vi "Graphic Test (2D picture speed).vi"() -> ()   [LabVIEW 2024]
panel:
  out "Other computation 2 Speed (Hz)":dbl
  out "Other computation Speed (Hz)":dbl
  out "Numeric":i32
  in  "stop":bool
  out "FPS":dbl
  out "PlayingScene":picture
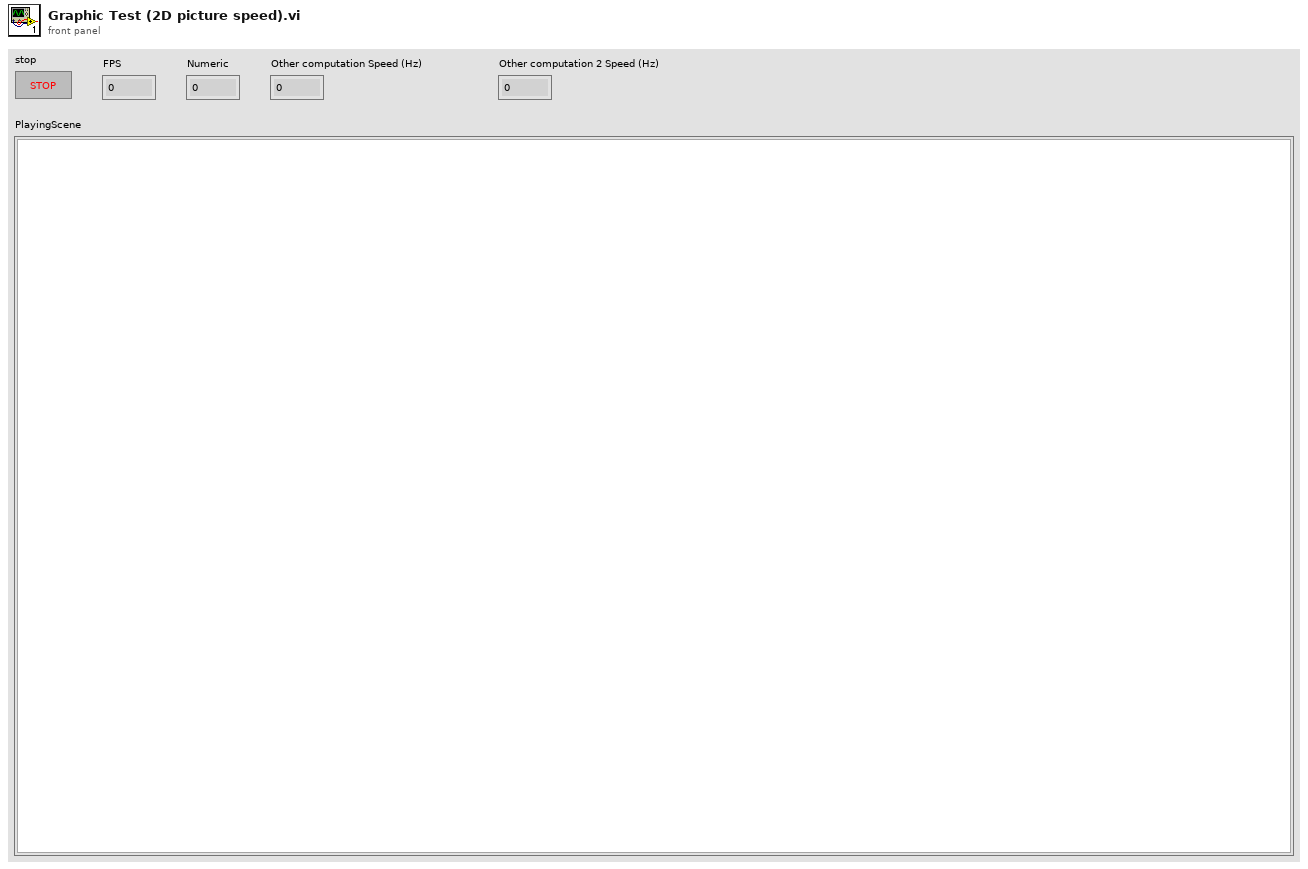
[diagram p1: front panel]
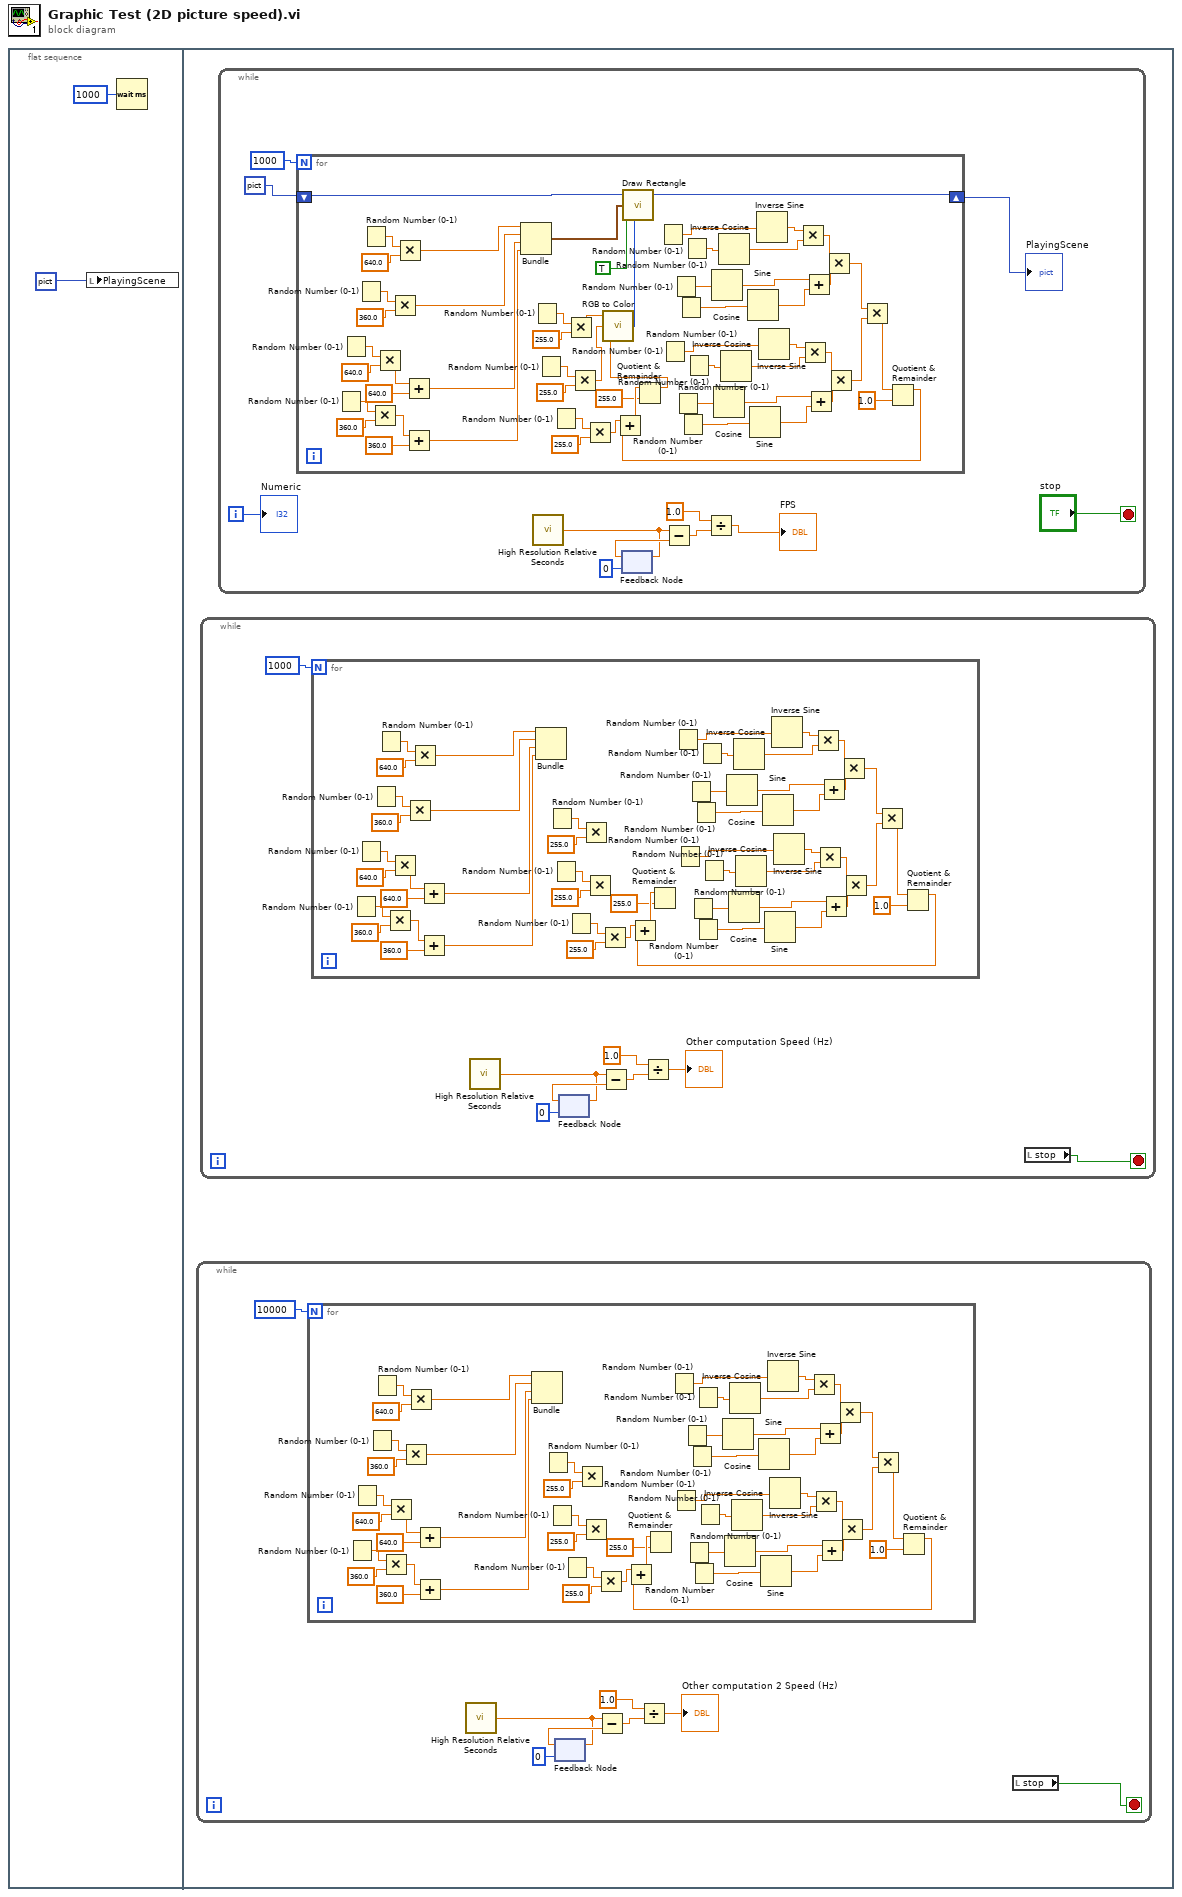
[diagram p0: block diagram]
diagram:
  n1 = flat-sequence {
    frame #0 {
      n2 = local write "PlayingScene"(picture data[5B] ("PlayingScene")) -> ()
      n3 = Wait (ms)(milliseconds to wait=u32 1000) -> ()  [unwired: 1 out]
    }
    frame #1 {
      n4 = while {
        stop <- w3 stop-if-true
        n5 = for {
          N: 10000 -> [_]
          n6 = Random Number (0-1)() -> (number: 0 to 1=w45:dbl)
          n7 = Random Number (0-1)() -> (number: 0 to 1=w47:dbl)
          n8 = Random Number (0-1)() -> (number: 0 to 1=w50:dbl)
          n9 = Random Number (0-1)() -> (number: 0 to 1=w53:dbl)
          n10 = Multiply(x=w45, y=360.0) -> (x*y=w41:dbl)
          n11 = Multiply(x=w47, y=640.0) -> (x*y=w44:dbl)
          n12 = Multiply(x=w50, y=360.0) -> (x*y=w49:dbl)
          n13 = Multiply(x=w53, y=640.0) -> (x*y=w52:dbl)
          n14 = Add(x=w44, y=640.0) -> (x+y=w43:dbl)
          n15 = Add(x=w41, y=360.0) -> (x+y=w42:dbl)
          n16 = Bundle(w52, w49, w43, w42) -> ()  [unwired: 1 in, 1 out]
          n17 = Random Number (0-1)() -> (number: 0 to 1=w59:dbl)
          n18 = Random Number (0-1)() -> (number: 0 to 1=w57:dbl)
          n19 = Random Number (0-1)() -> (number: 0 to 1=w55:dbl)
          n20 = Multiply(x=w59, y=255.0) -> ()  [unwired: 1 out]
          n21 = Multiply(x=w57, y=255.0) -> ()  [unwired: 1 out]
          n22 = Multiply(x=w55, y=255.0) -> (x*y=w26:dbl)
          n23 = Random Number (0-1)() -> (number: 0 to 1=w15:dbl)
          n24 = Random Number (0-1)() -> (number: 0 to 1=w30:dbl)
          n25 = Random Number (0-1)() -> (number: 0 to 1=w14:dbl)
          n26 = Random Number (0-1)() -> (number: 0 to 1=w29:dbl)
          n27 = Random Number (0-1)() -> (number: 0 to 1=w16:dbl)
          n28 = Random Number (0-1)() -> (number: 0 to 1=w31:dbl)
          n29 = Random Number (0-1)() -> (number: 0 to 1=w23:dbl)
          n30 = Random Number (0-1)() -> (number: 0 to 1=w38:dbl)
          n31 = Cosine(x=w14) -> (cos(x)=w20:dbl)
          n32 = Cosine(x=w29) -> (cos(x)=w35:dbl)
          n33 = Inverse Cosine(1:w23) -> (0:w21:dbl)
          n34 = Inverse Cosine(1:w38) -> (0:w36:dbl)
          n35 = Sine(x=w16) -> (sin(x)=w19:dbl)
          n36 = Sine(x=w31) -> (sin(x)=w34:dbl)
          n37 = Inverse Sine(1:w15) -> (0:w22:dbl)
          n38 = Inverse Sine(1:w30) -> (0:w37:dbl)
          n39 = Multiply(x=w22, y=w21) -> (x*y=w18:dbl)
          n40 = Multiply(x=w37, y=w36) -> (x*y=w33:dbl)
          n41 = Add(x=w20, y=w19) -> (x+y=w17:dbl)
          n42 = Add(x=w35, y=w34) -> (x+y=w32:dbl)
          n43 = Multiply(x=w18, y=w17) -> (x*y=w13:dbl)
          n44 = Multiply(x=w33, y=w32) -> (x*y=w12:dbl)
          n45 = Multiply(x=w13, y=w12) -> (x*y=w11:dbl)
          n46 = Quotient & Remainder(x=w11, y=1.0) -> (x-y*floor(x/y)=w27:dbl)  [unwired: 1 out]
          n47 = Add(x=w26, y=w27) -> (x+y=w25:dbl)
          n48 = Quotient & Remainder(x=w25, y=255.0) -> ()  [unwired: 2 out]
        }
        n49 = call <vilib>:"High Resolution Relative Seconds.vi"() -> ("relative seconds"=w5:dbl)
        n50 = feedback #1(u32 0 ("millisecond timer value")) -> (w6:dbl)
        n51 = feedback-in #1(w5) -> ()
        n52 = Subtract(x=w5, y=w6) -> (x-y=w9:dbl)
        n53 = Divide(x=1.0, y=w9) -> (x/y=→"Other computation 2 Speed (Hz)":dbl)
        n54 = local read "stop"() -> (w3:bool)
      }
      n55 = while {
        stop <- w67 stop-if-true
        n56 = for {
          N: 1000 -> [_]
          n57 = Random Number (0-1)() -> (number: 0 to 1=w103:dbl)
          n58 = Random Number (0-1)() -> (number: 0 to 1=w105:dbl)
          n59 = Random Number (0-1)() -> (number: 0 to 1=w108:dbl)
          n60 = Random Number (0-1)() -> (number: 0 to 1=w111:dbl)
          n61 = Multiply(x=w103, y=360.0) -> (x*y=w99:dbl)
          n62 = Multiply(x=w105, y=640.0) -> (x*y=w102:dbl)
          n63 = Multiply(x=w108, y=360.0) -> (x*y=w107:dbl)
          n64 = Multiply(x=w111, y=640.0) -> (x*y=w110:dbl)
          n65 = Add(x=w102, y=640.0) -> (x+y=w101:dbl)
          n66 = Add(x=w99, y=360.0) -> (x+y=w100:dbl)
          n67 = Bundle(w110, w107, w101, w100) -> ()  [unwired: 1 in, 1 out]
          n68 = Random Number (0-1)() -> (number: 0 to 1=w117:dbl)
          n69 = Random Number (0-1)() -> (number: 0 to 1=w115:dbl)
          n70 = Random Number (0-1)() -> (number: 0 to 1=w113:dbl)
          n71 = Multiply(x=w117, y=255.0) -> ()  [unwired: 1 out]
          n72 = Multiply(x=w115, y=255.0) -> ()  [unwired: 1 out]
          n73 = Multiply(x=w113, y=255.0) -> (x*y=w84:dbl)
          n74 = Random Number (0-1)() -> (number: 0 to 1=w73:dbl)
          n75 = Random Number (0-1)() -> (number: 0 to 1=w88:dbl)
          n76 = Random Number (0-1)() -> (number: 0 to 1=w72:dbl)
          n77 = Random Number (0-1)() -> (number: 0 to 1=w87:dbl)
          n78 = Random Number (0-1)() -> (number: 0 to 1=w74:dbl)
          n79 = Random Number (0-1)() -> (number: 0 to 1=w89:dbl)
          n80 = Random Number (0-1)() -> (number: 0 to 1=w81:dbl)
          n81 = Random Number (0-1)() -> (number: 0 to 1=w96:dbl)
          n82 = Cosine(x=w72) -> (cos(x)=w78:dbl)
          n83 = Cosine(x=w87) -> (cos(x)=w93:dbl)
          n84 = Inverse Cosine(1:w81) -> (0:w79:dbl)
          n85 = Inverse Cosine(1:w96) -> (0:w94:dbl)
          n86 = Sine(x=w74) -> (sin(x)=w77:dbl)
          n87 = Sine(x=w89) -> (sin(x)=w92:dbl)
          n88 = Inverse Sine(1:w73) -> (0:w80:dbl)
          n89 = Inverse Sine(1:w88) -> (0:w95:dbl)
          n90 = Multiply(x=w80, y=w79) -> (x*y=w76:dbl)
          n91 = Multiply(x=w95, y=w94) -> (x*y=w91:dbl)
          n92 = Add(x=w78, y=w77) -> (x+y=w75:dbl)
          n93 = Add(x=w93, y=w92) -> (x+y=w90:dbl)
          n94 = Multiply(x=w76, y=w75) -> (x*y=w71:dbl)
          n95 = Multiply(x=w91, y=w90) -> (x*y=w70:dbl)
          n96 = Multiply(x=w71, y=w70) -> (x*y=w69:dbl)
          n97 = Quotient & Remainder(x=w69, y=1.0) -> (x-y*floor(x/y)=w85:dbl)  [unwired: 1 out]
          n98 = Add(x=w84, y=w85) -> (x+y=w83:dbl)
          n99 = Quotient & Remainder(x=w83, y=255.0) -> ()  [unwired: 2 out]
        }
        n100 = call <vilib>:"High Resolution Relative Seconds.vi"() -> ("relative seconds"=w62:dbl)
        n101 = feedback #2(u32 0 ("millisecond timer value")) -> (w63:dbl)
        n102 = feedback-in #2(w62) -> ()
        n103 = Subtract(x=w62, y=w63) -> (x-y=w66:dbl)
        n104 = Divide(x=1.0, y=w66) -> (x/y=→"Other computation Speed (Hz)":dbl)
        n105 = local read "stop"() -> (w67:bool)
      }
      n106 = while {
        i -> [w119]
        stop <- "stop" stop-if-true
        n107 = for {
          N: 1000 -> [_]
          shift-right: [w185] -> w122
          shift-left: picture data[5B] ("PlayingScene") -> [w186]
          n108 = Random Number (0-1)() -> (number: 0 to 1=w165:dbl)
          n109 = Random Number (0-1)() -> (number: 0 to 1=w167:dbl)
          n110 = Random Number (0-1)() -> (number: 0 to 1=w170:dbl)
          n111 = Random Number (0-1)() -> (number: 0 to 1=w173:dbl)
          n112 = Multiply(x=w165, y=360.0) -> (x*y=w161:dbl)
          n113 = Multiply(x=w167, y=640.0) -> (x*y=w164:dbl)
          n114 = Multiply(x=w170, y=360.0) -> (x*y=w169:dbl)
          n115 = Multiply(x=w173, y=640.0) -> (x*y=w172:dbl)
          n116 = Add(x=w164, y=640.0) -> (x+y=w163:dbl)
          n117 = Add(x=w161, y=360.0) -> (x+y=w162:dbl)
          n118 = Bundle(w172, w169, w163, w162) -> (w175:cluster{dbl, dbl, dbl, dbl})  [unwired: 1 in]
          n119 = Random Number (0-1)() -> (number: 0 to 1=w182:dbl)
          n120 = Random Number (0-1)() -> (number: 0 to 1=w179:dbl)
          n121 = Random Number (0-1)() -> (number: 0 to 1=w177:dbl)
          n122 = Multiply(x=w182, y=255.0) -> (x*y=w181:dbl)
          n123 = Multiply(x=w179, y=255.0) -> (x*y=w176:dbl)
          n124 = Multiply(x=w177, y=255.0) -> (x*y=w146:dbl)
          n125 = Random Number (0-1)() -> (number: 0 to 1=w134:dbl)
          n126 = Random Number (0-1)() -> (number: 0 to 1=w150:dbl)
          n127 = Random Number (0-1)() -> (number: 0 to 1=w133:dbl)
          n128 = Random Number (0-1)() -> (number: 0 to 1=w149:dbl)
          n129 = Random Number (0-1)() -> (number: 0 to 1=w135:dbl)
          n130 = Random Number (0-1)() -> (number: 0 to 1=w151:dbl)
          n131 = Random Number (0-1)() -> (number: 0 to 1=w142:dbl)
          n132 = Random Number (0-1)() -> (number: 0 to 1=w158:dbl)
          n133 = Cosine(x=w133) -> (cos(x)=w139:dbl)
          n134 = Cosine(x=w149) -> (cos(x)=w155:dbl)
          n135 = Inverse Cosine(1:w142) -> (0:w140:dbl)
          n136 = Inverse Cosine(1:w158) -> (0:w156:dbl)
          n137 = Sine(x=w135) -> (sin(x)=w138:dbl)
          n138 = Sine(x=w151) -> (sin(x)=w154:dbl)
          n139 = Inverse Sine(1:w134) -> (0:w141:dbl)
          n140 = Inverse Sine(1:w150) -> (0:w157:dbl)
          n141 = Multiply(x=w141, y=w140) -> (x*y=w137:dbl)
          n142 = Multiply(x=w157, y=w156) -> (x*y=w153:dbl)
          n143 = Add(x=w139, y=w138) -> (x+y=w136:dbl)
          n144 = Add(x=w155, y=w154) -> (x+y=w152:dbl)
          n145 = Multiply(x=w137, y=w136) -> (x*y=w132:dbl)
          n146 = Multiply(x=w153, y=w152) -> (x*y=w131:dbl)
          n147 = Multiply(x=w132, y=w131) -> (x*y=w130:dbl)
          n148 = Quotient & Remainder(x=w130, y=1.0) -> (x-y*floor(x/y)=w147:dbl)  [unwired: 1 out]
          n149 = Add(x=w146, y=w147) -> (x+y=w145:dbl)
          n150 = Quotient & Remainder(x=w145, y=255.0) -> (x-y*floor(x/y)=w143:dbl)  [unwired: 1 out]
          n151 = call <vilib>:"RGB to Color.vi"("B"=w143, "G"=w176, "R"=w181) -> ("Color"=w184:u32)
          n152 = call <vilib>:"Draw Rectangle.vi"("picture"=w186, "rect"=w175, "fill?(F)"=TRUE, "color(black)"=w184) -> ("new picture"=w185:picture)  [unwired: 5 in]
        }
        "PlayingScene" <- w122
        n153 = call <vilib>:"High Resolution Relative Seconds.vi"() -> ("relative seconds"=w124:dbl)
        n154 = feedback-in #3(w124) -> ()
        n155 = feedback #3(u32 0 ("millisecond timer value")) -> (w125:dbl)
        n156 = Subtract(x=w124, y=w125) -> (x-y=w129:dbl)
        n157 = Divide(x=1.0, y=w129) -> (x/y=→"FPS":dbl)
        "Numeric" <- w119
      }
    }
  }
